vi "Write Animal.vi"(8 "error in (no error)":errorcluster, 10 "Animal.lvclass":refnum<class "Animal.lvclass">, 11 "Animal Test In":refnum<class "Animal Test.lvclass">) -> (0 "error out":errorcluster, 3 "Animal Test Out":refnum<class "Animal Test.lvclass">)   [LabVIEW 2020, in "Animal Test.lvclass"]
doc: "Write Animal"
uses:
  Animal Test.lvclass
  Animal Classes/Animal/Animal.lvclass
  Animal Test.lvclass/Animal Test.ctl
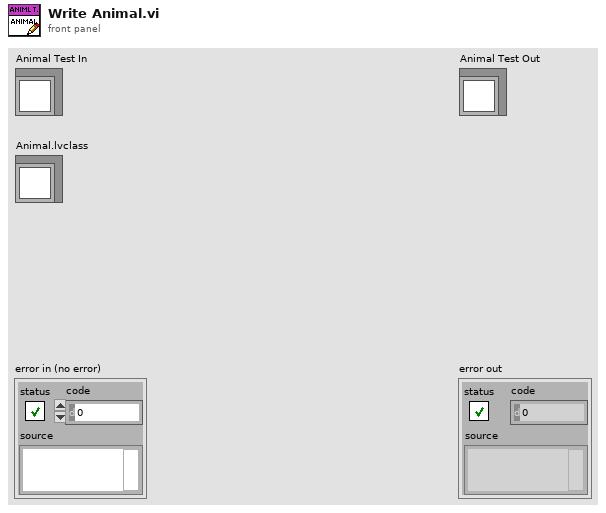
[diagram p1: front panel]
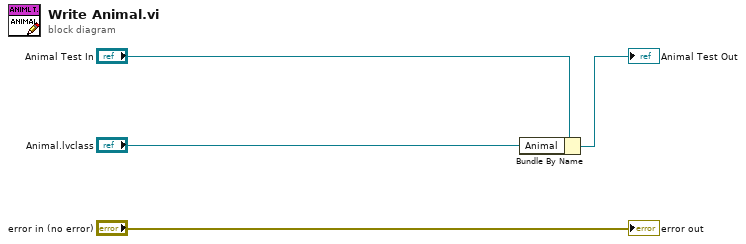
[diagram p0: block diagram]
diagram:
  n1 = Bundle By Name(cluster="Animal Test In", "Animal"="Animal.lvclass") -> (→"Animal Test Out":refnum<class "Animal Test.lvclass">)
  "error out" <- "error in (no error)"
